vi "STM Get Connection Reference (TCP).vi"(8 "error in":errorcluster, 11 "Connection Info":T1) -> (0 "error out":errorcluster, 2 "connection ID out":refnum<k5>, 3 "Connection Info":T1)   [LabVIEW 2015, in "Diagnostics Addon Engine.lvlib"]
doc: "Returns the TCP/IP connection reference."
uses:
  Diagnostics Addon Engine.lvlib
  stm_TCP Connection Info.ctl
  _SubVIs/stm_MetaDataElement.ctl
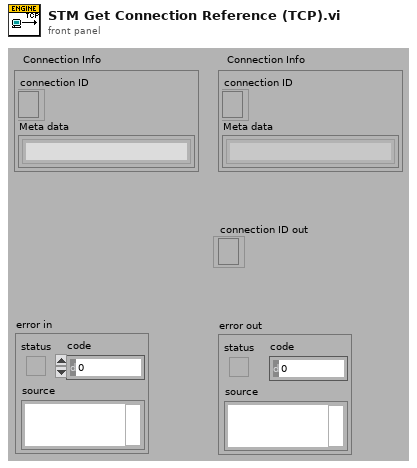
[diagram p1: front panel]
types:
  T1 = typedef "Diagnostics Addon Engine.lvlib/stm_TCP Connection Info.ctl" = cluster{"connection ID":refnum<k5>, "Meta data":T2[]}
  T2 = typedef "Diagnostics Addon Engine.lvlib/stm_MetaDataElement.ctl" = string
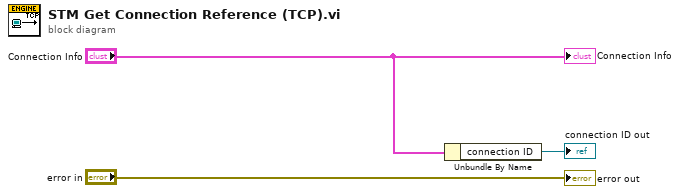
[diagram p0: block diagram]
diagram:
  n1 = Unbundle By Name("Connection Info") -> ("connection ID"=→"connection ID out":refnum<k5>)
  "Connection Info" <- "Connection Info"
  "error out" <- "error in"
